vi "Working Robot Car.vi"() -> ()   [LabVIEW 2016]
panel:
  in  "Turn Left Array 2":bool[](array[boolean]) caption="Turn Left"
  out "Boolean 4":bool
  out "Boolean":bool
  out "Boolean 2":bool
  out "Left IR":bool
  out "Voltage":dbl
  out "Middle IR":bool
  out "Voltage 2":dbl
  out "Right IR":bool
  out "Voltage 3":dbl
  out "Left IR Voltage":dynamicdata(graph)
  out "Mid IR Voltage":dynamicdata(graph)
  out "Right IR Voltage":dynamicdata(graph)
  out "Left PR (volts)":dbl
  out "Left PR Voltage":dynamicdata(graph)
  out "Mid PR (volts) 2":dbl
  out "Mid PR Voltage 2":dynamicdata(graph)
  out "Right PR (volts) 3":dbl
  out "Right PR Voltage 3":dynamicdata(graph)
  out "Left PR Black":bool
  out "Mid PR Black":bool
  out "Right PR Black":bool
  in  "Turn Right Array 2":bool[](array[boolean]) caption="Turn Right"
  in  "Forward Array 2":bool[](array[boolean]) caption="Forward"
  out "Boolean 6":bool
  out "Boolean 5":bool
  out "Boolean 3":bool
  in  "stop":bool
  # "NOTE: This is the final VI for your project. \nWhat you need to do is complete this template by\nadding the boolean (digital) logic on the back panel.\n(See block diagram)"
  # "Indicates if comparison on block diagram is true."
  # "Set your array values. For a value of 1, \nclick on the dot and make it turn black.\nFor a value of zero, leave the dot light gray"
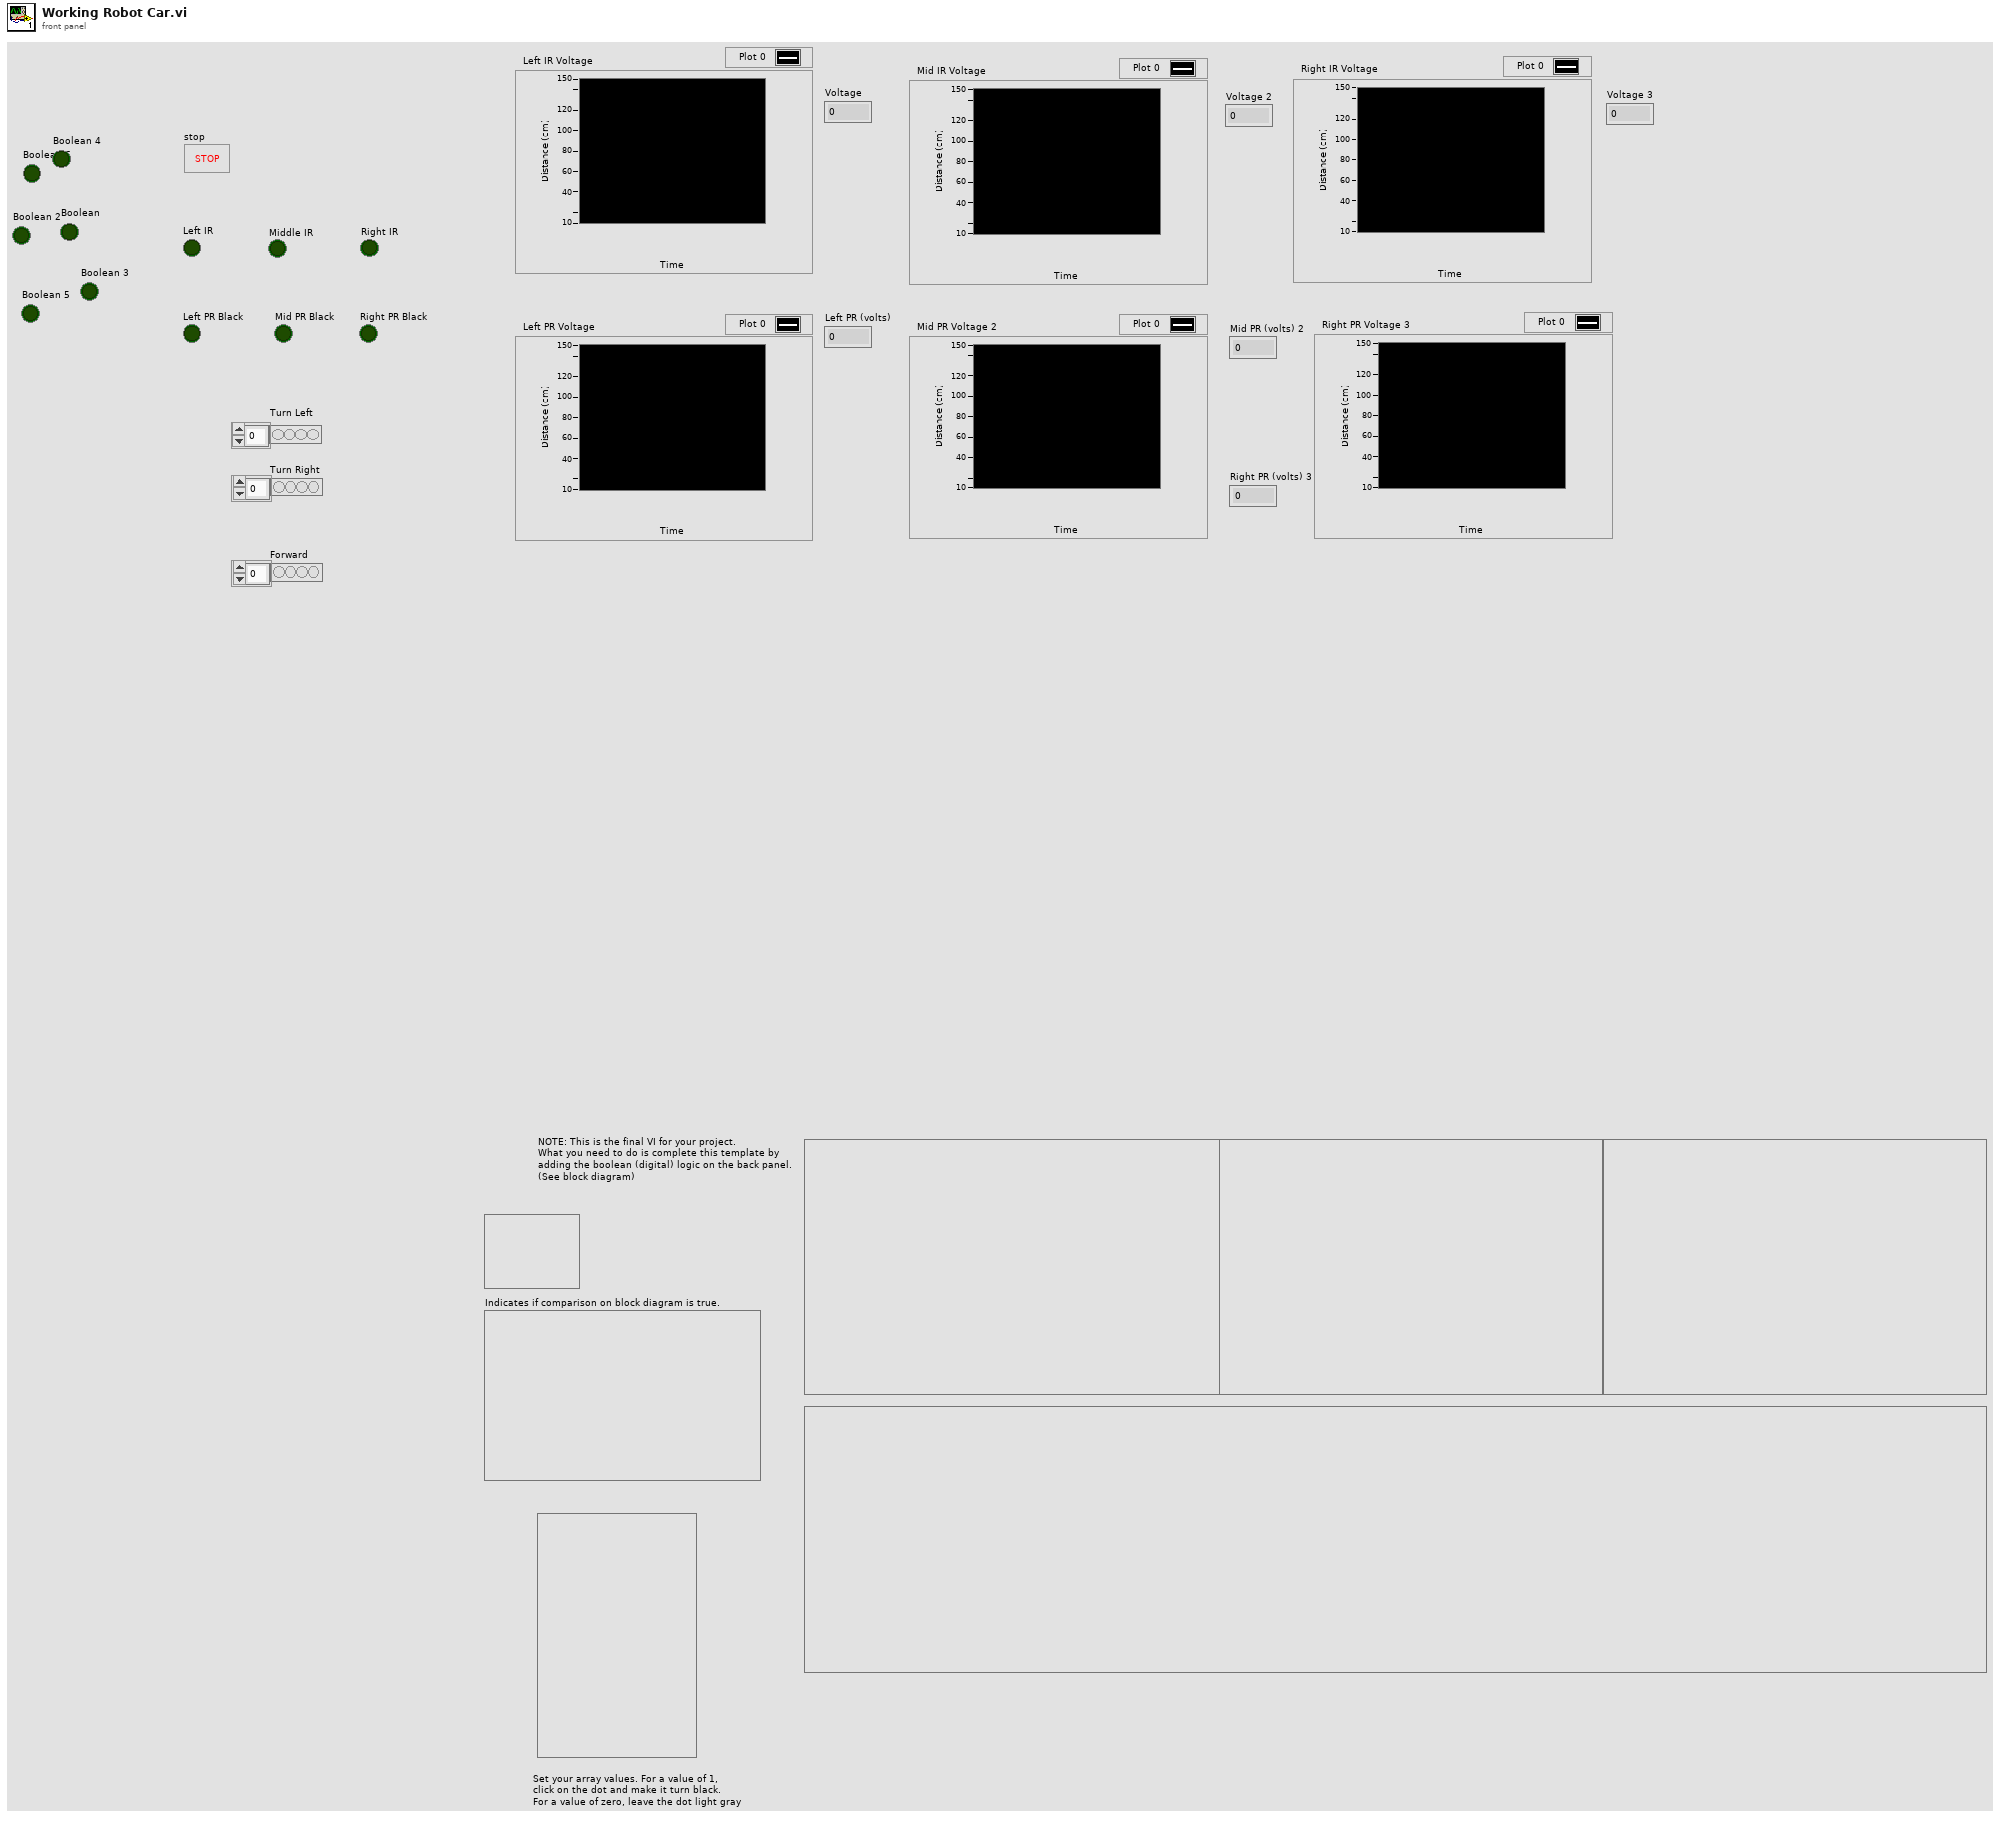
[diagram p1: front panel]
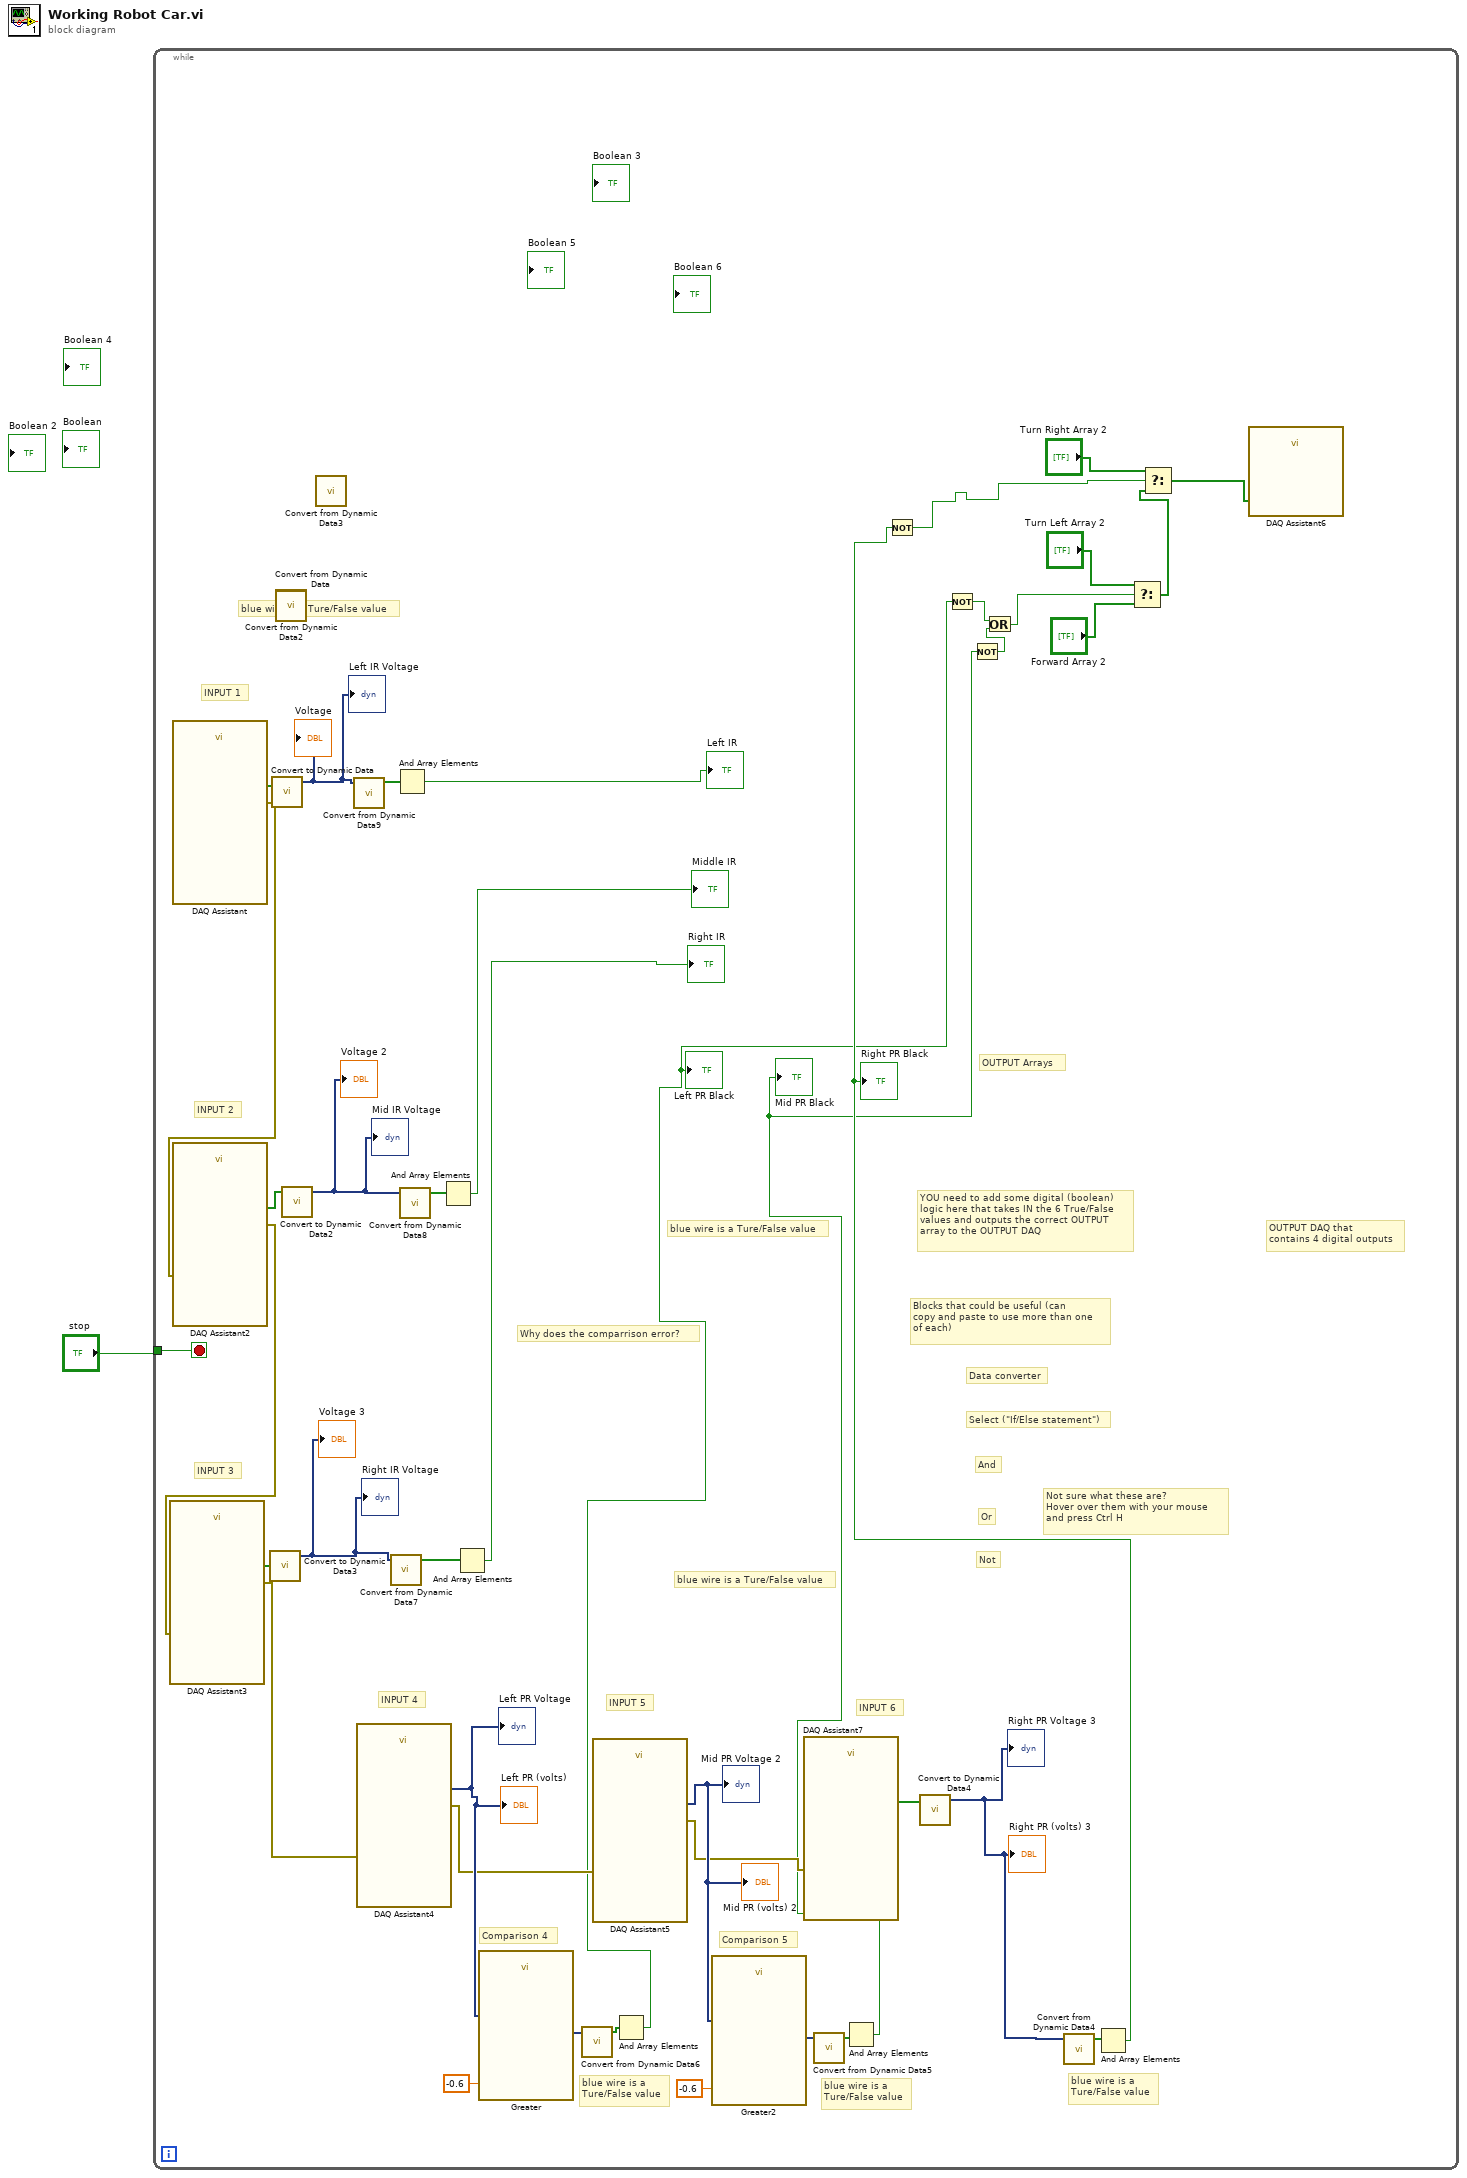
[diagram p0: block diagram]
diagram:
  n1 = while {
    tunnel: "stop" -> [w42]
    stop <- w42 stop-if-true
    # "Why does the comparrison error?"
    # "Not sure what these are? \nHover over them with your mouse\nand press Ctrl H"
    # "Not"
    # "Or"
    # "And"
    # "Select (\"If/Else statement\")"
    # "Data converter"
    # "Blocks that could be useful (can \ncopy and paste to use more than one\nof each)"
    # "YOU need to add some digital (boolean)\nlogic here that takes IN the 6 True/False \nvalues and outputs the correct OUTPUT \narray to the OUTPUT DAQ"
    # "blue wire is a \nTure/False value"
    # "blue wire is a\nTure/False value"
    # "blue wire is a \nTure/False value"
    # "blue wire is a Ture/False value"
    # "blue wire is a Ture/False value"
    # "blue wire is a Ture/False value"
    # "OUTPUT DAQ that\ncontains 4 digital outputs"
    # "OUTPUT Arrays"
    # "INPUT 6"
    # "Comparison 5"
    # "INPUT 5"
    # "Comparison 4"
    # "INPUT 4"
    # "INPUT 3"
    # "INPUT 2"
    # "INPUT 1"
    n2 = call "DAQ Assistant"() -> ("data"=w39:bool[], "error out"=w38:errorcluster)  [unwired: 17 in, 1 out]
    n3 = call "DAQ Assistant2"("error in"=w38) -> ("data"=w35:bool[], "error out"=w37:errorcluster)  [unwired: 16 in, 1 out]
    n4 = call "DAQ Assistant3"("error in"=w37) -> ("data"=w34:bool[], "error out"=w36:errorcluster)  [unwired: 16 in, 1 out]
    n5 = call "Convert to Dynamic Data3"("Array"=w34) -> ("Dynamic Data Type"=w24:dynamicdata)  [unwired: 3 in]
    "Voltage 3" <- w24
    "Right IR Voltage" <- w24
    n6 = call "Convert to Dynamic Data"("Array"=w39) -> ("Dynamic Data Type"=w18:dynamicdata)  [unwired: 3 in]
    "Voltage" <- w18
    "Left IR Voltage" <- w18
    n7 = call "Convert from Dynamic Data2"() -> ()  [unwired: 4 in, 1 out]
    n8 = call "Convert from Dynamic Data"() -> ()  [unwired: 4 in, 1 out]
    n9 = call "Convert to Dynamic Data2"("Array"=w35) -> ("Dynamic Data Type"=w21:dynamicdata)  [unwired: 3 in]
    "Voltage 2" <- w21
    "Mid IR Voltage" <- w21
    n10 = call "Convert from Dynamic Data3"() -> ()  [unwired: 4 in, 1 out]
    n11 = call "Convert from Dynamic Data9"("Dynamic Data Type"=w18) -> ("Array"=w17:bool[])  [unwired: 3 in]
    n12 = call "DAQ Assistant4"("error in"=w36) -> ("data"=w33:dynamicdata, "error out"=w32:errorcluster)  [unwired: 16 in, 1 out]
    "Left PR (volts)" <- w33
    "Left PR Voltage" <- w33
    n13 = call "Convert from Dynamic Data7"("Dynamic Data Type"=w24) -> ("Array"=w23:bool[])  [unwired: 3 in]
    n14 = And Array Elements(Boolean array=w17) -> (logical AND=→"Left IR":bool)
    n15 = call "Convert from Dynamic Data8"("Dynamic Data Type"=w21) -> ("Array"=w20:bool[])  [unwired: 3 in]
    n16 = And Array Elements(Boolean array=w20) -> (logical AND=→"Middle IR":bool)
    n17 = And Array Elements(Boolean array=w23) -> (logical AND=→"Right IR":bool)
    n18 = call "Greater"("Constant Value to Compare Against"=-0.6, "Operand 1"=w33) -> ("Result"=w26:dynamicdata)  [unwired: 8 in, 1 out]
    n19 = call "Convert from Dynamic Data6"("Dynamic Data Type"=w26) -> ("Array"=w25:bool[])  [unwired: 3 in]
    n20 = call "DAQ Assistant5"("error in"=w32) -> ("data"=w31:dynamicdata, "error out"=w15:errorcluster)  [unwired: 16 in, 1 out]
    "Mid PR (volts) 2" <- w31
    "Mid PR Voltage 2" <- w31
    n21 = And Array Elements(Boolean array=w25) -> (logical AND=w7:bool)
    "Left PR Black" <- w7
    n22 = call "Greater2"("Constant Value to Compare Against"=-0.6, "Operand 1"=w31) -> ("Result"=w28:dynamicdata)  [unwired: 8 in, 1 out]
    n23 = call "DAQ Assistant7"("error in"=w15) -> ("data"=w14:bool[])  [unwired: 16 in, 2 out]
    n24 = call "Convert from Dynamic Data5"("Dynamic Data Type"=w28) -> ("Array"=w27:bool[])  [unwired: 3 in]
    n25 = And Array Elements(Boolean array=w27) -> (logical AND=w2:bool)
    "Mid PR Black" <- w2
    n26 = call "Convert to Dynamic Data4"("Array"=w14) -> ("Dynamic Data Type"=w13:dynamicdata)  [unwired: 3 in]
    "Right PR (volts) 3" <- w13
    "Right PR Voltage 3" <- w13
    n27 = Not(x=w7) -> (.not. x?=w5:bool)
    n28 = Not(x=w2) -> (.not. x?=w3:bool)
    n29 = Or(x=w5, y=w3) -> (x .or. y?=w4:bool)
    n30 = call "Convert from Dynamic Data4"("Dynamic Data Type"=w13) -> ("Array"=w29:bool[])  [unwired: 3 in]
    n31 = And Array Elements(Boolean array=w29) -> (logical AND=w11:bool)
    "Right PR Black" <- w11
    n32 = Not(x=w11) -> (.not. x?=w6:bool)
    n33 = Select(t="Turn Left Array 2", s=w4, f="Forward Array 2") -> (s? t:f=w8:bool[])
    n34 = Select(t="Turn Right Array 2", s=w6, f=w8) -> (s? t:f=w30:bool[])
    n35 = call "DAQ Assistant6"("data"=w30) -> ()  [unwired: 17 in, 2 out]
  }
